vi "main.vi"(8 "error in (no error)":errorcluster, 10 "event":refnum<user-event>, 11 "functional":refnum<user-event>) -> (0 "error out":errorcluster)   [LabVIEW 2015, in "example_01.lvlib" / "interfaces.lvlib" / "dark.lvclass"]
uses:
  dark.lvclass
  functional/public/_controls/event_functional.ctl
  functional/public/_controls/event_functional_command.ctl
  functional/public/interface/_controls/event_data.ctl
  functional/public/interface/_controls/event_command.ctl
  functional/public/_controls/hmi_references.ctl
  functional/functional.lvlib
  functional/public/interface/interface.lvclass
panel:
  in  "do_it":bool
  out "random_number":dbl
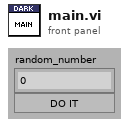
[diagram p1: front panel]
types:
  T1 = typedef "example_01.lvlib/functional.lvlib/event_functional_command.ctl" = enum16{"<command_functional>", "--high-level", "stop", "update_hmi_references", "load_interface", "--functional", "do_it", "<null>"}
  T2 = typedef "example_01.lvlib/functional.lvlib/hmi_references.ctl" = cluster{"vi_reference":refnum<vi>, "random_number":refnum<vi>, "do_it":refnum<vi>}
  T3 = typedef "example_01.lvlib/functional.lvlib/event_functional.ctl" = cluster{"command":T1, "data":variant}
  T4 = typedef "example_01.lvlib/functional.lvlib/interface.lvclass/event_command.ctl" = enum16{"<event_command>", "stop", "<null>"}
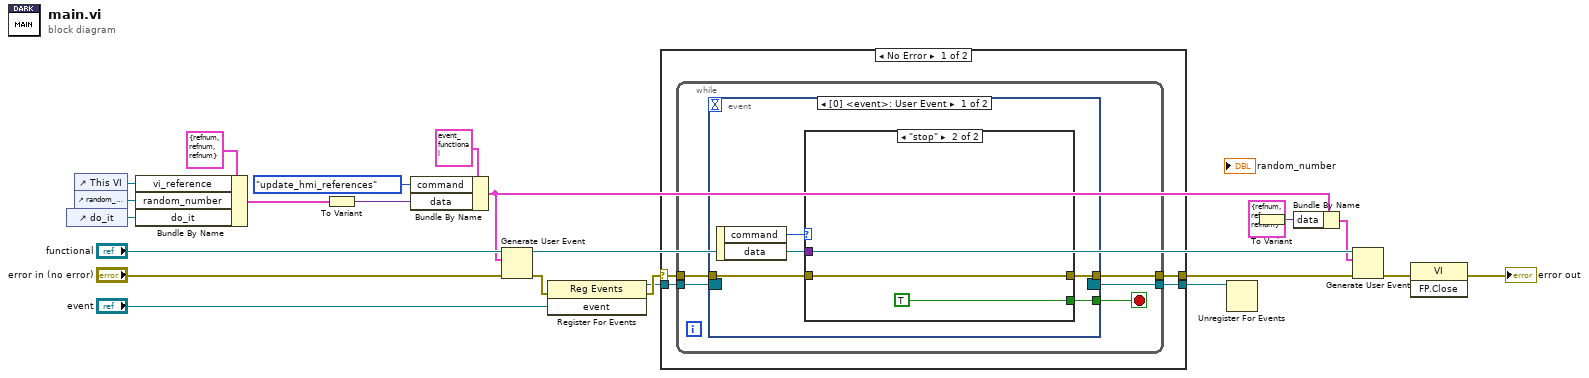
[diagram p0: block diagram]
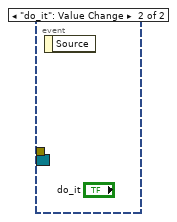
[diagram p3: hidden frame]
diagram:
  n1 = control-ref of="do_it"() -> (w20:refnum<vi>)
  n2 = control-ref of="This VI"() -> (w22:refnum<vi>)
  n3 = control-ref of="random_number"() -> (w21:refnum<vi>)
  n4 = Bundle By Name(cluster=T2 {"vi_reference"=refnum, "random_number"=refnum, "do_it"=refnum} ("hmi_references"), "vi_reference"=w22, "random_number"=w21, "do_it"=w20) -> (w16:T2)
  n5 = To Variant(anything=w16) -> (Variant=w15:variant)
  n6 = Bundle By Name(cluster=T3 {"command"=enum."<command_functional>", "data"=variant} ("event data"), "command"=event_functional_command."update_hmi_references", "data"=w15) -> (w11:T3)
  n7 = Generate User Event(user event="functional", event data cluster=w11, error in="error in (no error)") -> (user event out=w14:refnum<user-event>, error out=w7:errorcluster)  [unwired: 1 in]
  n8 = register-events(error in=w7, "event") -> (reference out=w5:refnum<event-registration>, error out=w6:errorcluster)  [unwired: 1 in]
  n9 = case shown="No Error" w6 {
    selector: w6 -> [w27 w42]
    tunnel: [w26 w42] -> w13
    tunnel: w5 -> [w25 w41]
    tunnel: [w24 w41] -> w4
    frame No Error {
      n10 = while {
        tunnel: w27 -> [w31]
        tunnel: [w30] -> w26
        tunnel: w25 -> [w29]
        tunnel: [w28] -> w24
        stop <- w32 stop-if-true
        n11 = event shown="[0] <event>: User Event" {
          selector: w29 -> [_ _]
          dyn-events: [_ _] -> w28
          timeout: _ -> [_ _]
          tunnel: [w34 _] -> w32
          tunnel: w31 -> [w36 _]
          tunnel: [w33 _] -> w30
          event User Event {
            n12 = event-data() -> ("command"=w37:T4, "data"=w35:variant)  [unwired: 1 in]
            n13 = case shown="\"stop\"" w37 {
              tunnel: w36 -> [w38 w39]
              tunnel: w35 -> [_ _]
              tunnel: [_ TRUE] -> w34
              tunnel: [w38 w39] -> w33
              frame Default {
              }
              frame "stop" {
              }
            }
          }
          event "do_it": Value Change {
            n14 = event-data() -> ()  [unwired: 1 in, 1 out]
          }
        }
      }
    }
    frame Error {
    }
  }
  n15 = Unregister For Events(event registration refnum=w4) -> ()  [unwired: 1 in, 1 out]
  n16 = To Variant(anything=T2 {"vi_reference"=refnum, "random_number"=refnum, "do_it"=refnum} ("hmi_references")) -> (Variant=w9:variant)
  n17 = Bundle By Name(cluster=w11, "data"=w9) -> (w10:T3)
  n18 = Generate User Event(user event=w14, event data cluster=w10, error in=w13) -> (error out=w3:errorcluster)  [unwired: 1 in, 1 out]
  n19 = invoke class="VI" method="FP.Close"(error in=w3) -> (error out=→"error out":errorcluster)  [unwired: 2 in, 2 out]
